vi "Volts to Tesla.vi"(1 "Calibration":T1={"Current Scale Factor kA/V"=1.0, "I->B"=[0.0, 1.0, 0.0], "B->I"=[0.0, 1.0, 0.0]} {"B->I" format="%.5e"; "Current Scale Factor kA/V" format="%.2f"; "I->B" format="%.5e"}, 2 "Console voltage":dbl=1.0 format="%.4f") -> (0 "Field":dbl=1.0 format="%.4f")   [LabVIEW 2019]
doc: "Converts a voltage from the magnet console output to tesla using the cubic fit from the constants K0, K1, K2. The voltage is first scaled to kA by a factor of 20.\nScott Hannahs, FBNML, May 1992"
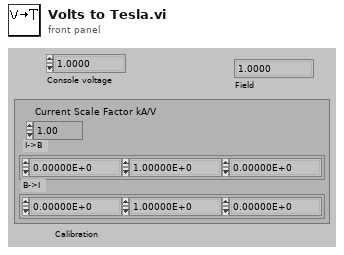
[diagram p1: front panel]
types:
  T1 = cluster{"Current Scale Factor kA/V":dbl, "I->B":dbl[], "B->I":dbl[]}
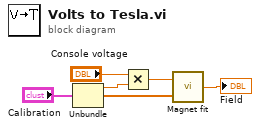
[diagram p0: block diagram]
diagram:
  n1 = Unbundle("Calibration") -> ("Current Scale Factor kA/V"=w4:dbl, "I->B"=w2:dbl[])  [unwired: 1 out]
  n2 = Multiply(x="Console voltage", y=w4) -> (x*y=w3:dbl)
  n3 = call "Magnet fit.vi"("Coefficients"=w2, "Magnet Parameter"=w3) -> ("Conjugate Parameter"=→"Field":dbl)
